vi "PLC.Debug.NewData.vi"(8 "error in (no error)":errorcluster, 10 "Data":T1={"Status"=0, "Ref1"="9998887770", "Serial1"="12345679", "Ref2"="", "Serial2"="", "Values"=[1.0, 2.0, 1.0, 1.0, 1.0, 4.0, 5.0, 1.0]} {"Values" format="%.3f"}, 11 "Idx":i32) -> (0 "error out":errorcluster, 2 "Saved":bool)   [LabVIEW 2016]
doc: "Connect to PLC\n\nWabco 2017 All right reserved\nAuthor: maciej.szupienko@wabco-auto.com"
uses:
  LowLevel/PLC.DataBlock.PLCvalues.ctl
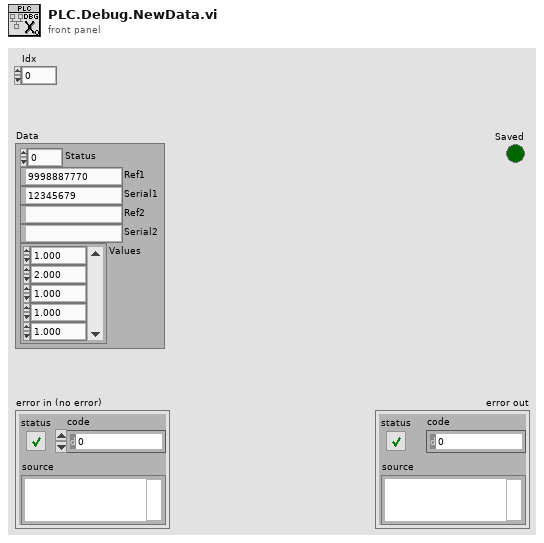
[diagram p1: front panel]
types:
  T1 = typedef "PLC.DataBlock.PLCvalues.ctl" = cluster{"Status":u8, "Ref1":string, "Serial1":string, "Ref2":string, "Serial2":string, "Values":sgl[]}
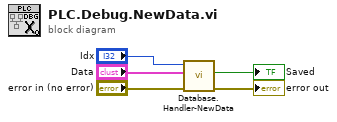
[diagram p0: block diagram]
diagram:
  n1 = call "Database.Handler-NewData.vi"("error in"="error in (no error)", "Data"="Data", "Idx"="Idx") -> ("error out"=→"error out":errorcluster, "Saved"=→"Saved":bool)  [unwired: 7 in]
